vi "FABR-Plot Metrics.vi"(0 "Analysis":T1, 1 "I-O":refnum<vi>, 11 "error in (no error)":errorcluster) -> (15 "error out":errorcluster)   [LabVIEW 2020]
uses:
  Typedefs/FABR-Analysis State.ctl
panel:
  # "Freq X Level X Time"
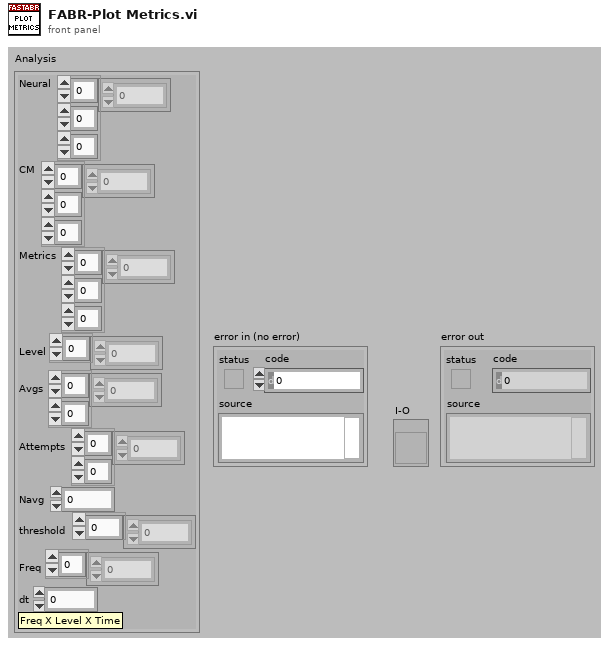
[diagram p1: front panel]
types:
  T1 = typedef "FABR-Analysis State.ctl" = cluster{"Neural":dbl[][][], "CM":dbl[][][], "Metrics":dbl[][][], "Level":dbl[], "Avgs":i32[][], "Attempts":i32[][], "Navg":i32, "threshold":dbl[], "Freq":dbl[], "dt":dbl}
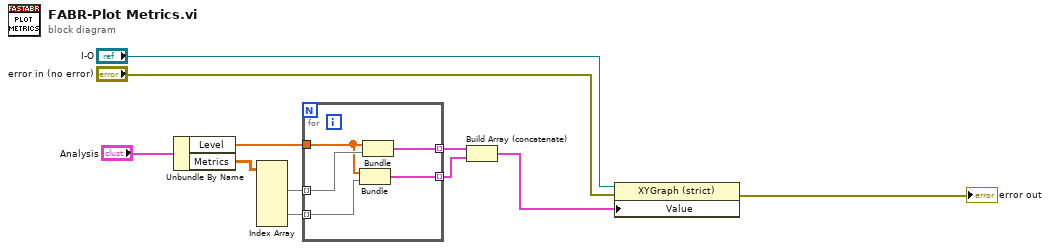
[diagram p0: block diagram]
diagram:
  n1 = Unbundle By Name("Analysis") -> ("Level"=w10:dbl[], "Metrics"=w6:dbl[][][])
  n2 = Index Array(array=w6) -> (element #1=w5:dbl[][], element #2=w4:dbl[][])  [unwired: 6 in]
  n3 = for {
    tunnel: w10 -> [w13]
    tunnel: w5 -> [w15] mode=indexing
    tunnel: [w16] -> w3 mode=indexing
    tunnel: w4 -> [w14] mode=indexing
    tunnel: [w12] -> w2 mode=indexing
    n4 = Bundle("Level"=w13, "Metrics"=w14) -> (w12:cluster{"Level":dbl[], "Metrics":dbl[]})  [unwired: 1 in]
    n5 = Bundle("Level"=w13, "Metrics"=w15) -> (w16:cluster{"Level":dbl[], "Metrics":dbl[]})  [unwired: 1 in]
  }
  n6 = Build Array (concatenate)(w3, w2) -> (w1:cluster{"Level":dbl[], "Metrics":dbl[]}[])
  n7 = property class="XYGraph (strict)"(reference="I-O", error in="error in (no error)", "Value"=w1) -> (error out=→"error out":errorcluster)  [unwired: 1 out]
